vi "Initialize Hardware.vi"(8 "error in":errorcluster, 9 "reset (F)":bool, 10 "set board to system time (F)":bool, 11 "board identifier in":u8) -> (0 "error out":errorcluster, 2 "module handle out":u8, 3 "board identifier out":u8)   [LabVIEW 2020, in "AIM ARINC 429 Hardware API.lvlib"]
uses:
  AIM ARINC 429 Hardware API.lvlib
  <instrlib>/AIM GmbH/ARINC-429/Controls/HwManager_action.ctl
  074549ee-7c0c-4d09-9718-ca6b598eb695.vi
  <instrlib>/AIM GmbH/ARINC-429/subvi/Error Converter (ErrCode or Status).vi
  <instrlib>/AIM GmbH/ARINC-429/subvi/Get Library Path.vi
  <instrlib>/AIM GmbH/ARINC-429/VIs/Library/Api429Lib Error Desc Get.vi
  <instrlib>/AIM GmbH/ARINC-429/subvi/Get Error Number Offset.vi
  <vilib>/Utility/error.llb/Error Cluster From Error Code.vi
  <instrlib>/AIM GmbH/ARINC-429/AIM429LV.lvlib
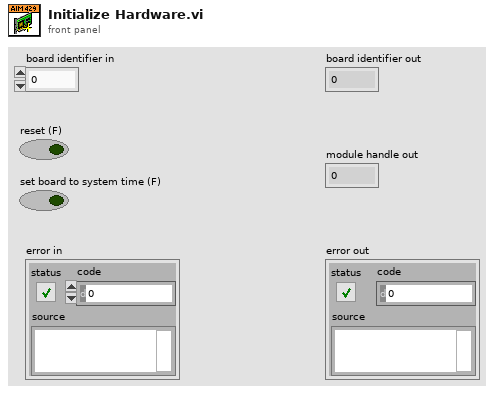
[diagram p1: front panel]
types:
  T1 = typedef "AIM429LV.lvlib/HwManager_action.ctl" = enum16{"Get Resource", "Remove Instance", "Add Resource", "Clear All", "Remove Resource"}
  T2 = cluster{"day":u32, "hour":u32, "minute":u32, "second":u32, "millisecond":u32}
  T3 = typedef "LVDateTimeRec.ctl" = cluster{"fractional second":dbl, "second":i32, "minute":i32, "hour":i32, "day of month":i32, "month":i32, "year":i32, "day of week":i32, "day of year":i32, "DST":i32}
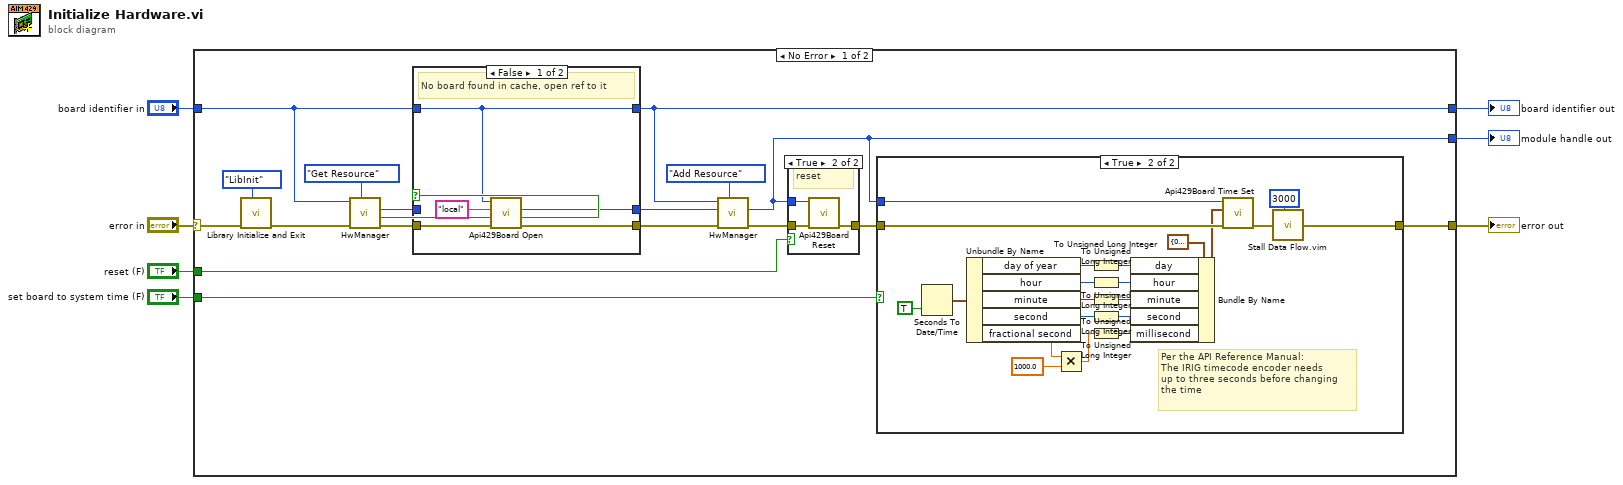
[diagram p0: block diagram]
diagram:
  n1 = case shown="No Error" "error in" {
    selector: "error in" -> [w16 w60]
    tunnel: [w9 _] -> w7
    tunnel: [w8 w60] -> w6
    tunnel: "reset (F)" -> [w25 _]
    tunnel: "board identifier in" -> [w13 w61]
    tunnel: [w12 w61] -> w2
    tunnel: "set board to system time (F)" -> [w11 _]
    frame No Error {
      n2 = call "Library Initialize and Exit.vi"("action"=enum16{"LibInit", "LibExit"}."LibInit", "error in"=w16) -> ("error out"=w14:errorcluster)  [unwired: 7 in, 2 out]
      n3 = call <instrlib>:"HwManager.vi"("Action (Get)"=HwManager_action."Get Resource", "error in (no error)"=w14, "board id"=w13) -> ("error out"=w17:errorcluster, "found"=w18:bool, "module handle out"=w19:u8)  [unwired: 5 in, 1 out]
      n4 = case shown="False" w18 {
        tunnel: w17 -> [w55 w58]
        tunnel: w13 -> [w52 w57]
        tunnel: [w54 w58] -> w22
        tunnel: [w53 w59] -> w23
        tunnel: w19 -> [_ w59]
        tunnel: [w52 w57] -> w12
        frame False {
          # "No board found in cache, open ref to it"
          n5 = call <instrlib>:"Api429Board Open.vi"("error in (no error)"=w55, "ac_SrvName"="local" ("ServerName"), "board_id"=w52) -> ("error out"=w54:errorcluster, "handle out"=w53:u8)  [unwired: 7 in]
        }
        frame True {
          # "Board Found"
        }
      }
      n6 = call <instrlib>:"HwManager.vi"("Action (Get)"=HwManager_action."Add Resource", "error in (no error)"=w22, "module handle in"=w23, "board id"=w12) -> ("error out"=w24:errorcluster, "module handle out"=w9:u8)  [unwired: 4 in, 2 out]
      n7 = case shown="True" w25 {
        tunnel: [w48 w49] -> w10
        tunnel: w24 -> [w48 w51]
        tunnel: w9 -> [_ w50]
        frame False {
          # "continue"
        }
        frame True {
          # "reset"
          n8 = call <instrlib>:"Api429Board Reset.vi"("error in (no error)"=w51, "board_handle"=w50) -> ("error out"=w49:errorcluster)  [unwired: 9 in]
        }
      }
      n9 = case shown="True" w11 {
        tunnel: w10 -> [w26 w32]
        tunnel: w9 -> [_ w30]
        tunnel: [w26 w27] -> w8
        frame False {
        }
        frame True {
          # "Per the API Reference Manual:\nThe IRIG timecode encoder needs\nup to three seconds before changing\nthe time"
          n10 = Seconds To Date/Time(to UTC (F)=TRUE) -> (date time rec=w47:T3)  [unwired: 1 in]
          n11 = Unbundle By Name(w47) -> ("day of year"=w46:i32, "hour"=w45:i32, "minute"=w44:i32, "second"=w43:i32, "fractional second"=w38:dbl)
          n12 = Multiply(x=w38, y=1000.0) -> (x*y=w37:dbl)
          n13 = To Unsigned Long Integer(number=w46) -> (unsigned 32bit integer=w42:u32)
          n14 = To Unsigned Long Integer(number=w45) -> (unsigned 32bit integer=w41:u32)
          n15 = To Unsigned Long Integer(number=w44) -> (unsigned 32bit integer=w40:u32)
          n16 = To Unsigned Long Integer(number=w43) -> (unsigned 32bit integer=w39:u32)
          n17 = To Unsigned Long Integer(number=w37) -> (unsigned 32bit integer=w36:u32)
          n18 = Bundle By Name(cluster=T2 {"day"=0, "hour"=0, "minute"=0, "second"=0, "millisecond"=0} ("irig_time"), "day"=w42, "hour"=w41, "minute"=w40, "second"=w39, "millisecond"=w36) -> (w31:T2)
          n19 = call <instrlib>:"Api429Board Time Set.vi"("error in (no error)"=w32, "irig_time"=w31, "board_handle"=w30) -> ("error out"=w29:errorcluster)  [unwired: 8 in]
          n20 = call "Stall Data Flow.vim"("value in"=w29, "milliseconds to wait"=u32 3000) -> ("value out"=w27:errorcluster)  [unwired: 1 out]
        }
      }
    }
    frame Error {
    }
  }
  "module handle out" <- w7
  "error out" <- w6
  "board identifier out" <- w2
